vi "add.volume.vi"(7 "folder map in":map{i32, map{string, i32}}(c390), 8 "error in (no error)":errorcluster, 10 "Path":path, 11 "volume map in":map{i32, T1}(c390)) -> (0 "error out":errorcluster, 3 "volume map out":map{i32, T1}(c390), 5 "folder map out":map{i32, map{string, i32}}(c390))   [LabVIEW 2024, in "manager_daemon.lvclass"]
uses:
  manager_daemon.lvclass
  type_defs/VolumeData--cluster.ctl
  CV_Shared_Library/volume.type--enum.ctl
  manager_daemon.lvclass/manager_daemon.ctl
  CV_Shared_Library/CV_Shared_Library.lvlib
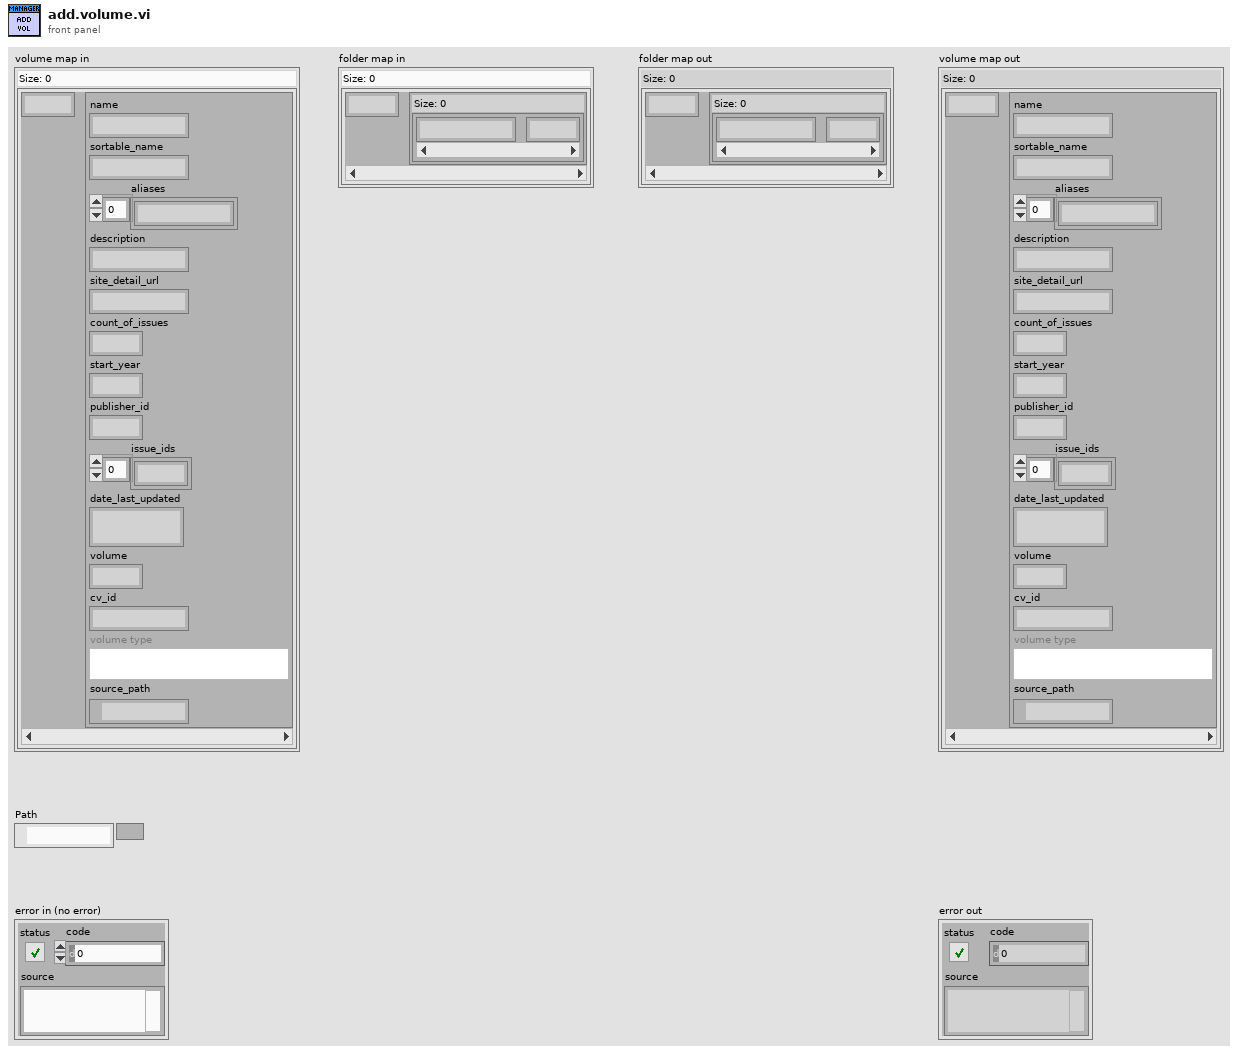
[diagram p1: front panel]
types:
  T1 = typedef "manager_daemon.lvclass/VolumeData--cluster.ctl" = cluster{"name":string, "sortable_name":string, "aliases":string[], "description":string, "site_detail_url":string, "count_of_issues":i32, "start_year":i32, "publisher_id":i32, "issue_ids":i32[], "date_last_updated":timestamp, "volume":i32, "cv_id":string, "volume type":T2, "source_path":path}
  T2 = typedef "CV_Shared_Library.lvlib/volume.type--enum.ctl" = enum16{"Ongoing", "Limited Series", "Annual", "One Shot", "Reprint/Document", "Star Comics", "Epic Comics"}
  T3 = typedef "CV_RESTful_Lib.lvlib/local_volume--cluster.ctl" = cluster{"id":i32, "name":string, "sortable_name":string, "aliases":string[], "description":string, "site_detail_url":string, "count_of_issues":i32, "start_year":i32, "publisher_id":i32, "issue_ids":i32[], "date_last_updated":timestamp, "volume":i32, "cv_id":string, "volume type":T2}
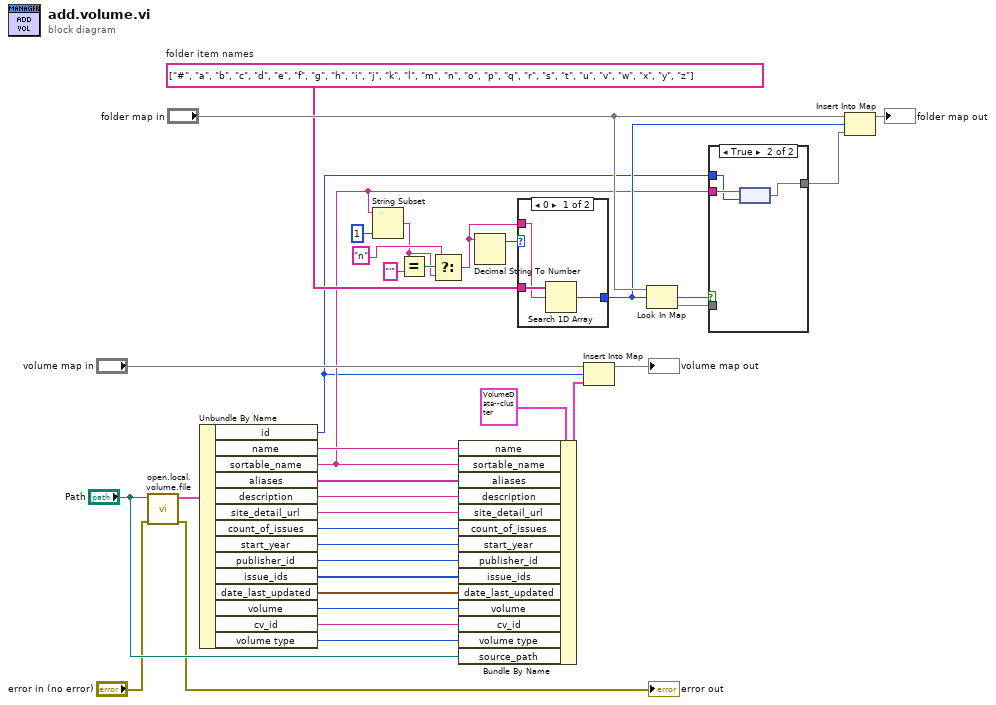
[diagram p0: block diagram]
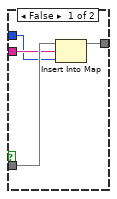
[diagram p2: hidden frame]
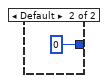
[diagram p3: hidden frame]
diagram:
  w4 = string[] ["#", "a", "b", "c", "d", "e", "f", "g", "h", "i", "j", "k", "l", "m", "n", "o", "p", "q", "r", "s", "t", "u", "v", "w", "x", "y", "z"]  # folder item names
  n1 = call "open.local.volume.file.vi"("error in (no error)"="error in (no error)", "volume json"="Path") -> ("error out"=→"error out":errorcluster, "volume"=w18:T3)  [unwired: 8 in]
  n2 = Unbundle By Name(w18) -> ("id"=w2:i32, "name"=w19:string, "sortable_name"=w3:string, "aliases"=w20:string[], "description"=w21:string, "site_detail_url"=w22:string, "count_of_issues"=w23:i32, "start_year"=w24:i32, "publisher_id"=w25:i32, "issue_ids"=w26:i32[], "date_last_updated"=w27:timestamp, "volume"=w28:i32, "cv_id"=w29:string, "volume type"=w30:T2)
  n3 = String Subset(string=w3, length (rest)=1 ("length (rest)")) -> (substring=w10:string)  [unwired: 1 in]
  n4 = Equal?(x=w10, y="'" ("x")) -> (x = y?=w12:bool)
  n5 = Select(t="n" ("x"), s=w12, f=w10) -> (s? t:f=w9:string)
  n6 = Bundle By Name(cluster=T1 {"name"="", "sortable_name"="", "aliases"=[], "description"="", "site_detail_url"="", "count_of_issues"=0, "start_year"=0, "publisher_id"=0, "issue_ids"=[], "date_last_updated"=timestamp(0 s since 1904-01-01), "volume"=0, "cv_id"="", "volume type"=enum."Ongoing", "source_path"=path ""} ("value"), "name"=w19, "sortable_name"=w3, "aliases"=w20, "description"=w21, "site_detail_url"=w22, "count_of_issues"=w23, "start_year"=w24, "publisher_id"=w25, "issue_ids"=w26, "date_last_updated"=w27, "volume"=w28, "cv_id"=w29, "volume type"=w30, "source_path"="Path") -> (w32:T1)
  n7 = Decimal String To Number(string=w9) -> (offset past number=w15:i32)  [unwired: 2 in, 1 out]
  n8 = case shown="0" w15 {
    tunnel: w9 -> [w38 _]
    tunnel: w4 -> [w39 _]
    tunnel: [w37 0 ("index of element")] -> w6
    frame 0 {
      n9 = Search 1D Array(1D array=w39, element=w38) -> (index of element=w37:i32)  [unwired: 1 in]
    }
    frame Default {
    }
  }
  n10 = Insert Into Map(map in="volume map in", key=w2, value=w32) -> (map out=→"volume map out":map{i32, T1})  [unwired: 2 out]
  n11 = Look In Map(map="folder map in", key=w6) -> (key not found?=w8:bool, value=w7:map{string, i32})  [unwired: 1 in]
  n12 = case shown="True" w8 {
    tunnel: w7 -> [w44 _]
    tunnel: w3 -> [w43 w47]
    tunnel: w2 -> [w42 w46]
    tunnel: [w41 w45] -> w5
    frame False {
      n13 = Insert Into Map(map in=w44, key=w43, value=w42) -> (map out=w41:map{string, i32})  [unwired: 2 out]
    }
    frame True {
      n14 = node(w47, w46) -> (w45:map{string, i32})
    }
  }
  n15 = Insert Into Map(map in="folder map in", key=w6, value=w5) -> (map out=→"folder map out":map{i32, map{string, i32}})  [unwired: 2 out]
